vi "Scale_Graph_X (SubVI).vi"(9 "Array":dbl[](array[numeric]), 10 "Übersetzung ermitteln aus":u8, 11 "XYGraph (Eingang)":refnum<vi>) -> ()   [LabVIEW 2014]
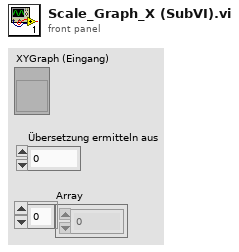
[diagram p1: front panel]
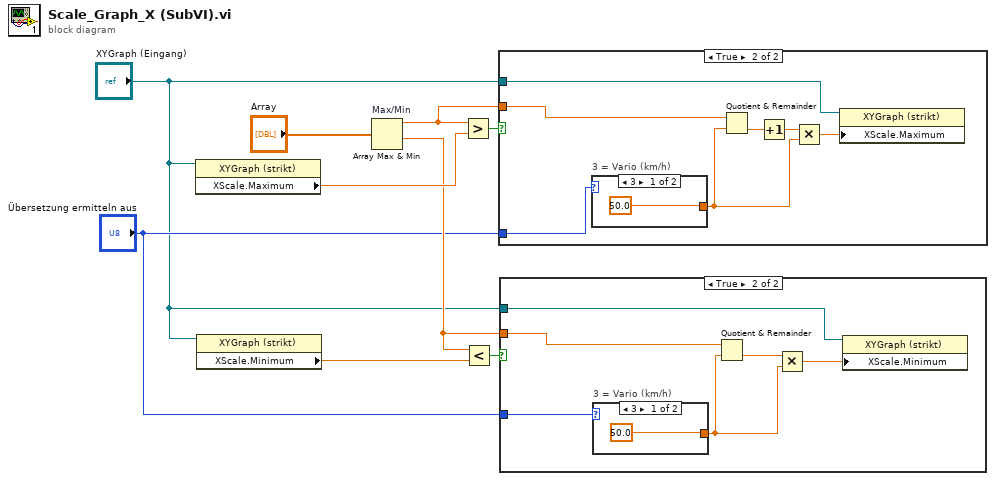
[diagram p0: block diagram]
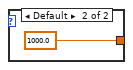
[diagram p3: hidden frame]
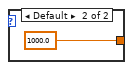
[diagram p5: hidden frame]
diagram:
  n1 = property on="Eigenschaftsknoten" class="XYGraph (strikt)"(reference="XYGraph (Eingang)") -> ("XScale.Maximum"=w6:dbl)  [unwired: 1 in, 2 out]
  n2 = property on="Eigenschaftsknoten" class="XYGraph (strikt)"(reference="XYGraph (Eingang)") -> ("XScale.Minimum"=w4:dbl)  [unwired: 1 in, 2 out]
  n3 = Array Max & Min "Max/Min"(array="Array") -> (max value=w7:dbl, min value=w3:dbl)  [unwired: 2 out]
  n4 = Greater?(x=w7, y=w6) -> (0:w8:bool)
  n5 = Less?(x=w3, y=w4) -> (x < y?=w5:bool)
  n6 = case shown="True" w8 {
    tunnel: w7 -> [_ w12]
    tunnel: "XYGraph (Eingang)" -> [_ w14]
    tunnel: "Übersetzung ermitteln aus" -> [_ w10]
    frame False {
    }
    frame True {
      n7 = case "3 = Vario (km/h)" shown="3" w10 {
        tunnel: [50.0 1000.0] -> w11
        frame 3 {
        }
        frame Default {
        }
      }
      n8 = Quotient & Remainder(x=w12, y=w11) -> (floor(x/y)=w15:dbl)  [unwired: 1 out]
      n9 = Increment(x=w15) -> (x+1=w16:dbl)
      n10 = Multiply(x=w16, y=w11) -> (x*y=w13:dbl)
      n11 = property on="Eigenschaftsknoten" class="XYGraph (strikt)"(reference=w14, "XScale.Maximum"=w13) -> ()  [unwired: 1 in, 2 out]
    }
  }
  n12 = case shown="True" w5 {
    tunnel: w3 -> [_ w23]
    tunnel: "XYGraph (Eingang)" -> [_ w24]
    tunnel: "Übersetzung ermitteln aus" -> [_ w21]
    frame False {
    }
    frame True {
      n13 = case "3 = Vario (km/h)" shown="3" w21 {
        tunnel: [50.0 1000.0] -> w22
        frame 3 {
        }
        frame Default {
        }
      }
      n14 = Quotient & Remainder(x=w23, y=w22) -> (floor(x/y)=w20:dbl)  [unwired: 1 out]
      n15 = Multiply(x=w20, y=w22) -> (x*y=w19:dbl)
      n16 = property on="Eigenschaftsknoten" class="XYGraph (strikt)"(reference=w24, "XScale.Minimum"=w19) -> ()  [unwired: 1 in, 2 out]
    }
  }
